vi "Change Waveform.vi"(8 "error in":errorcluster, 10 "Waveforms UI Ctrl Ref":T2, 11 "Waveform Meas Config Ctrl Ref":T1) -> (0 "error out":errorcluster)   [LabVIEW 2025, in "Fgen Script Mode UI.lvlib"]
uses:
  Fgen Script Mode UI.lvlib
  Typedef/Waveforms UI Ctrl Ref.ctl
  Typedef/Waveform Meas Config Ctrl Ref.ctl
  Typedef/Wfm Typedef.ctl
panel:
  in  "Auto Name?":bool=TRUE
  in  "Wfm Name in Script":string
  in  "Waveform Selection":i32(listbox)
  out "Selected Waveform Preview":waveform(dbl)(graph)
  in  "File Path":path
  in  "Cancel":bool
  in  "OK":bool
  # "* After configure the TDMS file path, select one waveform from the Waveform Selection to add and press OK."
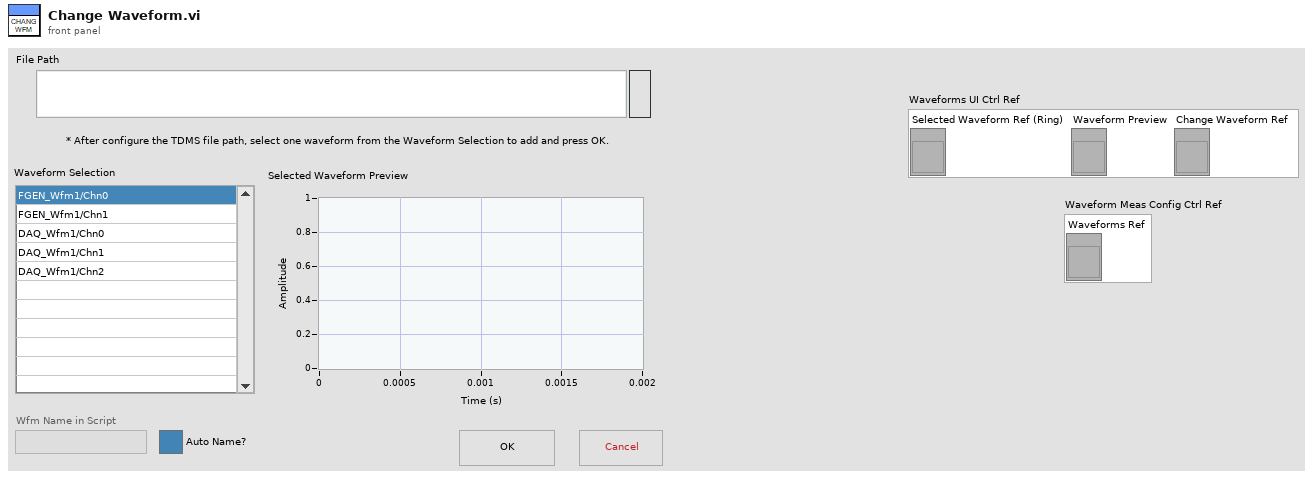
[diagram p1: front panel]
types:
  T1 = typedef "Fgen Script Mode UI.lvlib/Waveform Meas Config Ctrl Ref.ctl" = cluster{"Waveforms Ref":refnum<vi>}
  T2 = typedef "Fgen Script Mode UI.lvlib/Waveforms UI Ctrl Ref.ctl" = cluster{"Selected Waveform Ref (Ring)":refnum<vi>, "Waveform Preview":refnum<vi>, "Change Waveform Ref":refnum<vi>}
  T3 = typedef "Fgen Script Mode UI.lvlib/Wfm Typedef.ctl" = cluster{"Name":string, "Path":string, "Grp":string, "Chn":string}
  T4 = enum8{"Enabled", "Disabled", "Disabled and Grayed Out"}
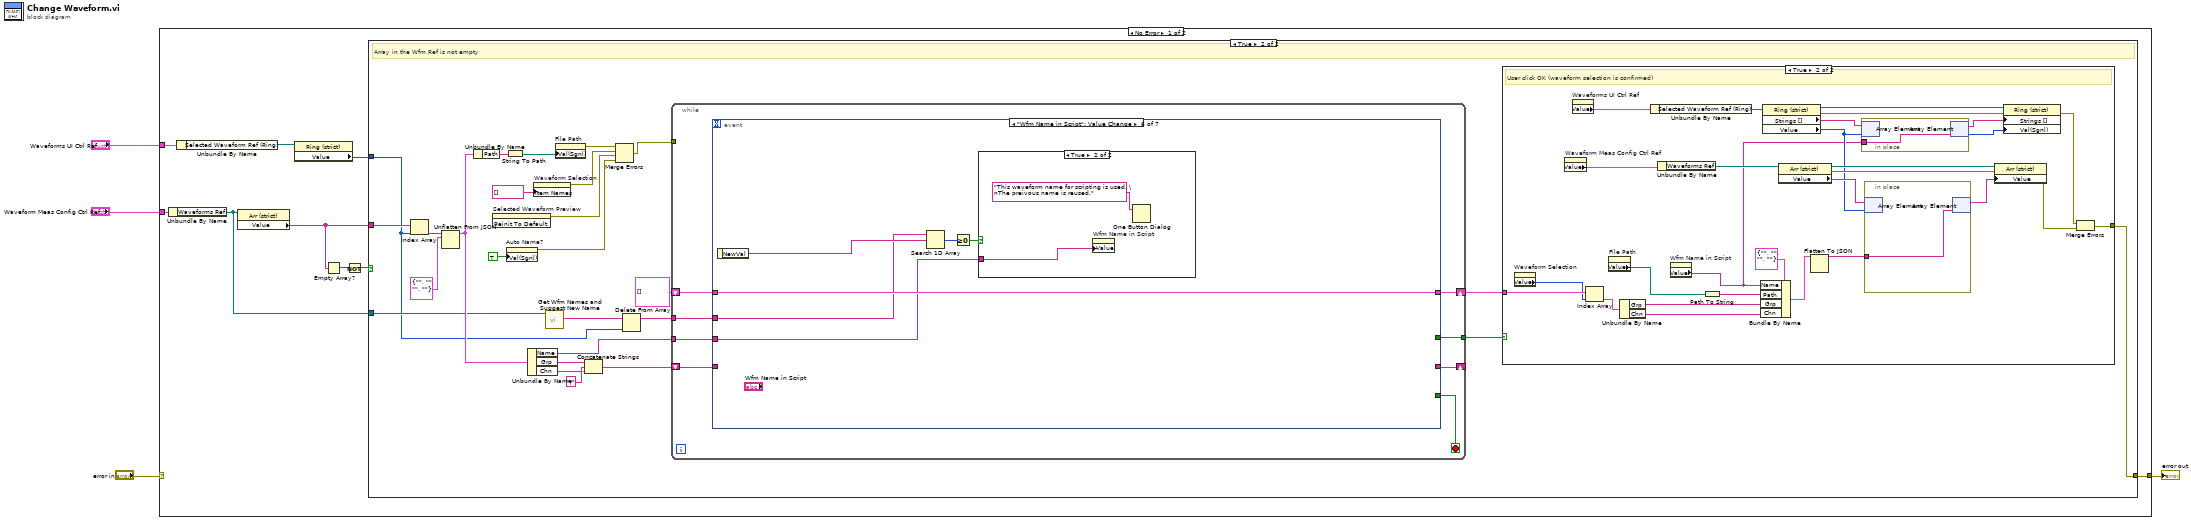
[diagram p0: block diagram]
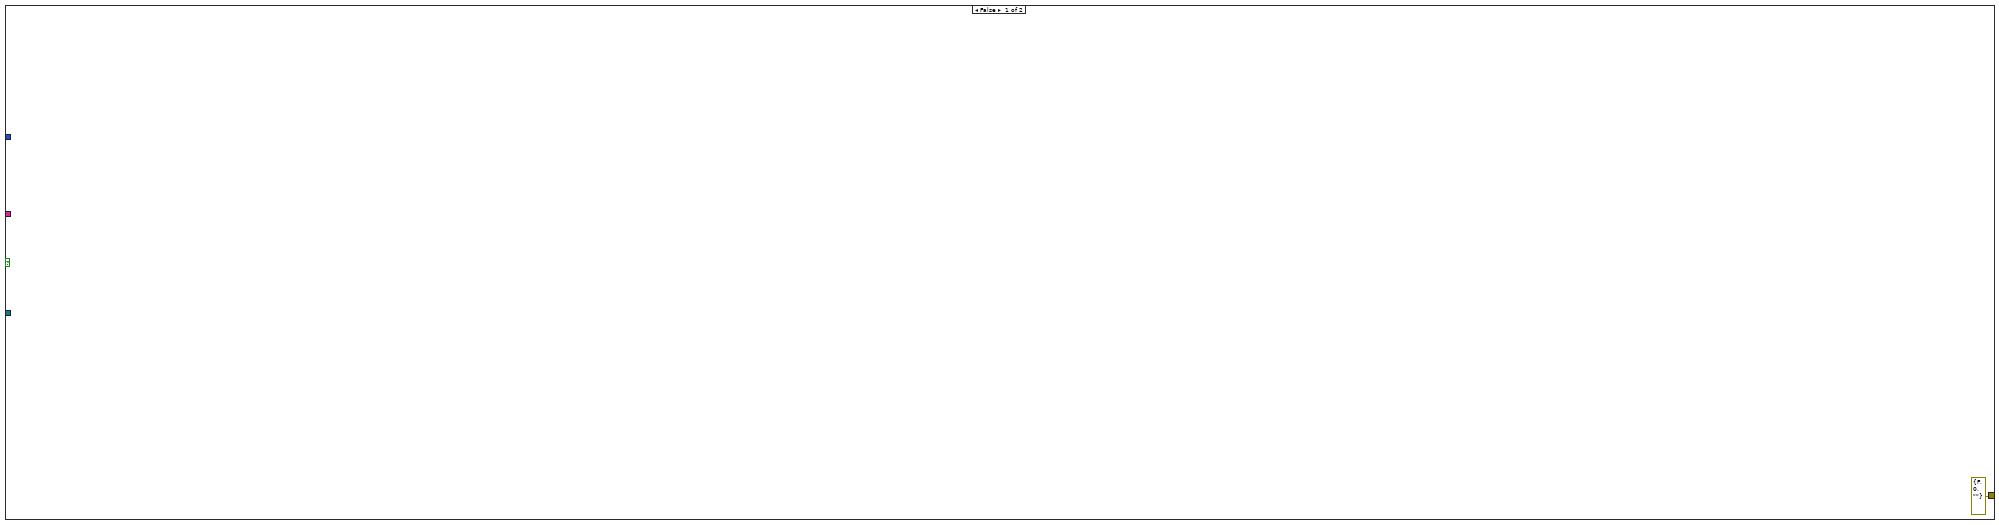
[diagram p2: hidden frame]
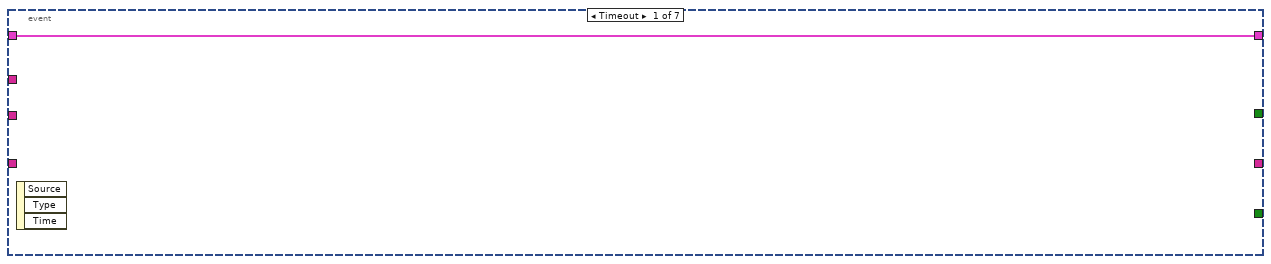
[diagram p4: hidden frame]
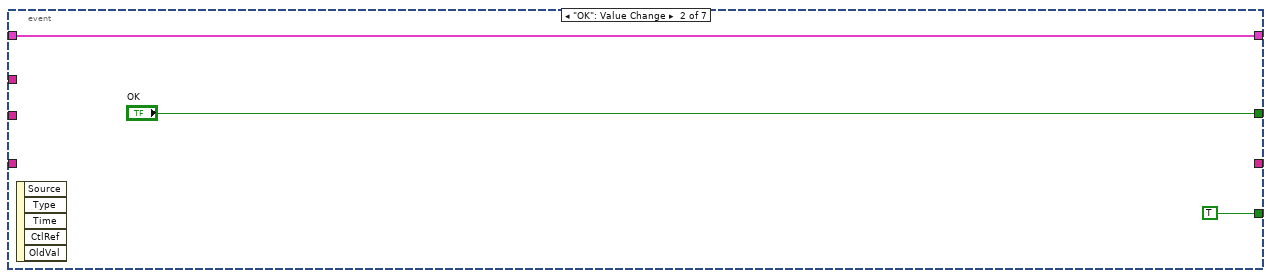
[diagram p5: hidden frame]
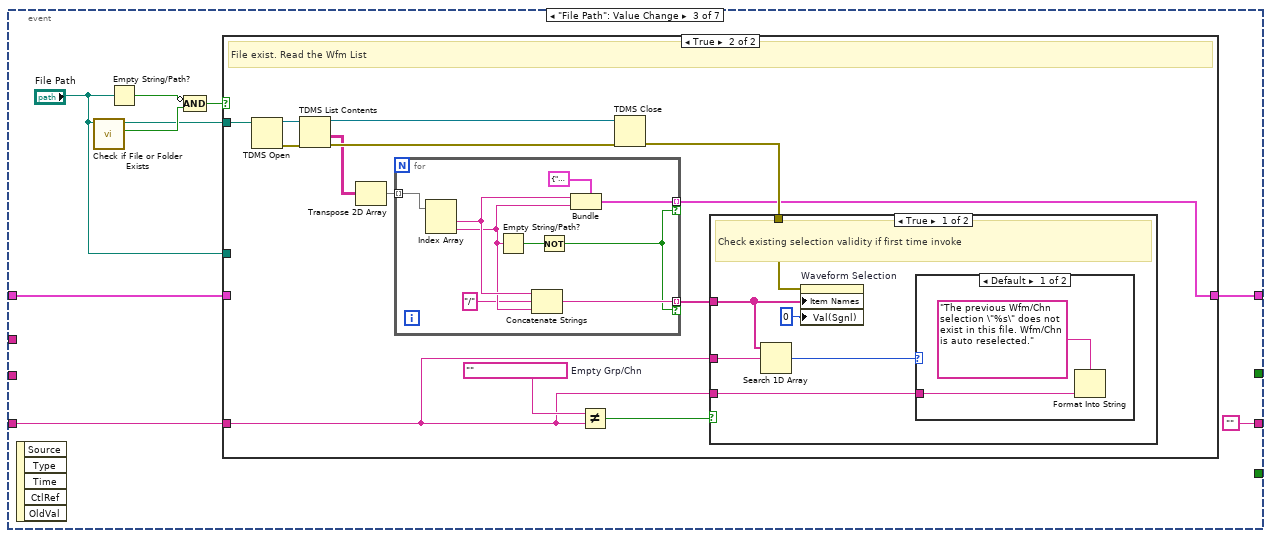
[diagram p6: hidden frame]
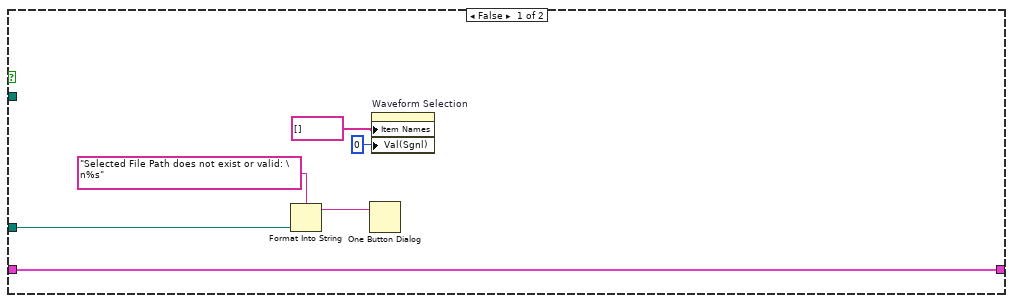
[diagram p7: hidden frame]
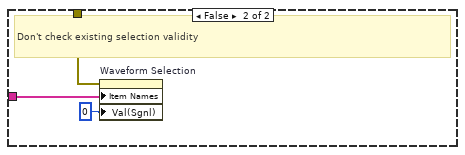
[diagram p9: hidden frame]
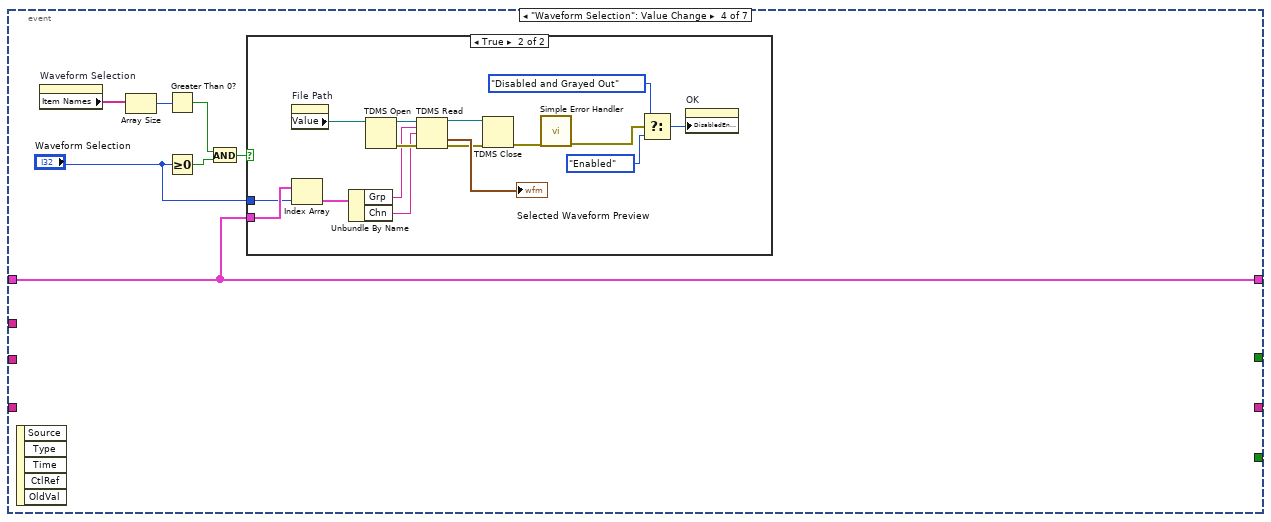
[diagram p10: hidden frame]
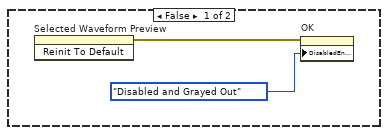
[diagram p11: hidden frame]
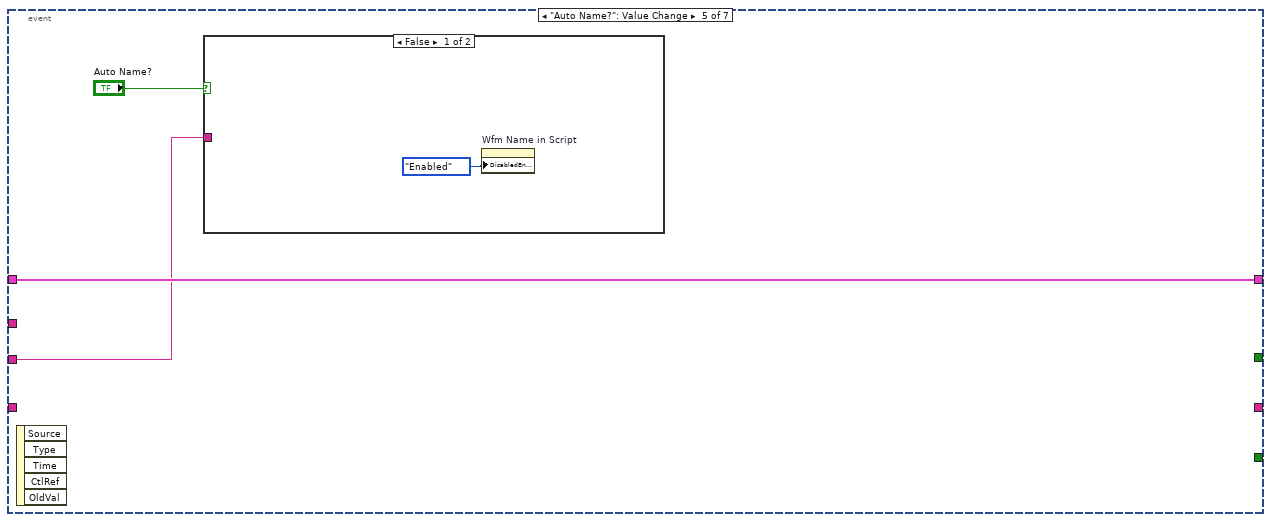
[diagram p12: hidden frame]
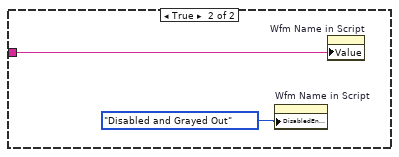
[diagram p13: hidden frame]
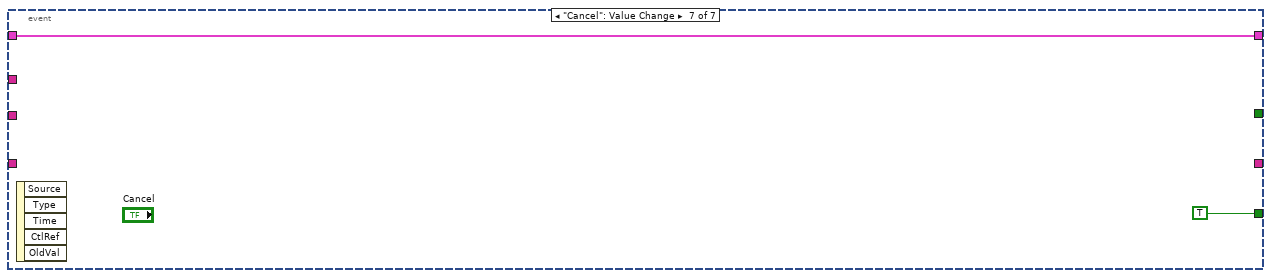
[diagram p15: hidden frame]
diagram:
  n1 = case shown="No Error" "error in" {
    selector: "error in" -> [_ w172]
    tunnel: [w13 w172] -> w3
    tunnel: "Waveforms UI Ctrl Ref" -> [w12 _]
    tunnel: "Waveform Meas Config Ctrl Ref" -> [w10 _]
    frame No Error {
      n2 = Unbundle By Name(w10) -> ("Waveforms Ref"=w7:refnum<vi>)
      n3 = Unbundle By Name(w12) -> ("Selected Waveform Ref (Ring)"=w11:refnum<vi>)
      n4 = property class="Arr (strict)"(reference=w7) -> ("Value"=w9:string[])  [unwired: 1 in, 2 out]
      n5 = property class="Ring (strict)"(reference=w11) -> ("Value"=w6:u16)  [unwired: 1 in, 2 out]
      n6 = Empty Array?(array=w9) -> (empty?=w8:bool)
      n7 = Not(x=w8) -> (.not. x?=w5:bool)
      n8 = case shown="True" w5 {
        tunnel: [errorcluster {"status"=FALSE, "code"=0, "source"=""} ("error IO") w32] -> w13
        tunnel: w9 -> [_ w29]
        tunnel: w7 -> [_ w19]
        tunnel: w6 -> [_ w17]
        frame False {
        }
        frame True {
          # "Array in the Wfm Ref is not empty"
          n9 = Index Array(array=w29, index=w17) -> (element=w27:string)
          n10 = Unflatten From JSON(JSON string=w27, type and defaults=T3 {"Name"="", "Path"="", "Grp"="", "Chn"=""} ("Waveform")) -> (value=w24:T3)  [unwired: 5 in, 1 out]
          n11 = Unbundle By Name(w24) -> ("Path"=w26:string)
          n12 = invoke on="Selected Waveform Preview" class="WFGraph (strict)" method="Reinit To Default"() -> (error out=w35:errorcluster)  [unwired: 3 in, 2 out]
          n13 = String To Path(string=w26) -> (path=w25:path)
          n14 = property on="Auto Name?" class="Bool (strict)"("Val(Sgnl)"=TRUE ("Value (Signaling)")) -> (error out=w31:errorcluster)  [unwired: 2 in, 1 out]
          n15 = Unbundle By Name(w24) -> ("Name"=w15:string, "Grp"=w22:string, "Chn"=w21:string)
          n16 = property on="Waveform Selection" class="LstBox (strict)"("Item Names"=string[] []) -> (error out=w36:errorcluster)  [unwired: 2 in, 1 out]
          n17 = call "Get Wfm Names and Suggest New Name.vi"("Wfm Ref In"=w19) -> ("Wfm Names"=w18:string[])  [unwired: 7 in, 3 out]
          n18 = property on="File Path" class="Path"("Val(Sgnl)"=w25) -> (error out=w39:errorcluster)  [unwired: 2 in, 1 out]
          n19 = Concatenate Strings(w22, "/" ("string"), w21) -> (w20:string)
          n20 = Merge Errors(w39, w36, w35, w31) -> (w37:errorcluster)
          n21 = Delete From Array(array=w18, index=w17) -> (array with subset deleted=w16:string[])  [unwired: 1 in, 1 out]
          n22 = while {
            tunnel: w37 -> [_]
            shift-right: [w77] -> w33
            shift-left: cluster{"Grp":string, "Chn":string}[] [] -> [w76]
            tunnel: [w75] -> w34
            shift-right: [w73] -> _
            shift-left: w20 -> [w74]
            tunnel: w16 -> [w72]
            tunnel: w15 -> [w71]
            stop <- w78 stop-if-true
            n23 = event shown="[5] \"Wfm Name in Script\": Value Change" {
              selector: _ -> [_ _ _ _ _ _ _]
              dyn-events: _ -> [_ _ _ _ _ _ _]
              timeout: _ -> [_ _ _ _ _ _ _]
              tunnel: [_ "OK" _ _ _ _ _] -> w75
              tunnel: [_ TRUE _ _ _ _ TRUE] -> w78
              tunnel: [w79 w80 w87 w132 w158 w167 w170] -> w77
              tunnel: w76 -> [w79 w80 w86 w132 w158 w167 w170]
              tunnel: w74 -> [_ _ w84 _ _ _ _]
              tunnel: [_ _ "" _ _ _ _] -> w73
              tunnel: w72 -> [_ _ _ _ _ w162 _]
              tunnel: w71 -> [_ _ _ _ w156 w163 _]
              event Timeout {
                n24 = event-data() -> ()  [unwired: 1 in, 3 out]
              }
              event "OK": Value Change {
                n25 = event-data() -> ()  [unwired: 1 in, 5 out]
              }
              event "File Path": Value Change {
                n26 = event-data() -> ()  [unwired: 1 in, 5 out]
                n27 = call <vilib>:"Check if File or Folder Exists.vi"("path"="File Path") -> ("file or folder exists?"=w90:bool, "dup path"=w88:path)  [unwired: 8 in, 1 out]
                n28 = Empty String/Path?(string/path="File Path") -> (empty?=w91:bool)
                n29 = Compound Arithmetic op=AND(invert w91, w90) -> (w89:bool)
                n30 = case shown="True" w89 {
                  tunnel: w88 -> [_ w110]
                  tunnel: [w97 w101] -> w87
                  tunnel: w86 -> [w97 _]
                  tunnel: "File Path" -> [w92 _]
                  tunnel: w84 -> [_ w98]
                  frame False {
                    n31 = Format Into String(format string="Selected File Path does not exist or valid: \n%s" ("message"), w92) -> (resulting string=w94:string)  [unwired: 2 in, 1 out]
                    n32 = One Button Dialog(message=w94) -> ()  [unwired: 1 in, 1 out]
                    n33 = property on="Waveform Selection" class="LstBox (strict)"("Item Names"=string[] [], "Val(Sgnl)"=0 ("Waveform Selection")) -> ()  [unwired: 2 in, 2 out]
                  }
                  frame True {
                    w100 = ""  # Empty Grp/Chn
                    # "File exist. Read the Wfm List"
                    n34 = TDMS Open(11:w110) -> (0:w109:errorcluster, 3:w108:refnum<k34>)  [unwired: 6 in]
                    n35 = TDMS List Contents(4:w109, 7:w108) -> (0:w106:errorcluster, 1:w104:string[][], 3:w107:refnum<k34>)  [unwired: 1 in, 1 out]
                    n36 = Transpose 2D Array(2D array=w104) -> (transposed array=w105:string[][])
                    n37 = for {
                      tunnel: w105 -> [w130] mode=indexing
                      tunnel: [w127] -> w101 mode=indexing if=w122
                      tunnel: [w123] -> w103 mode=indexing if=w122
                      n38 = Index Array(array=w130) -> (element #1=w126:string, element #2=w125:string)  [unwired: 2 in]
                      n39 = Empty String/Path?(string/path=w125) -> (empty?=w129:bool)
                      n40 = Concatenate Strings(w126, "/" ("string"), w125) -> (w123:string)
                      n41 = Not(x=w129) -> (.not. x?=w122:bool)
                      n42 = Bundle(cluster=cluster{"Grp":string, "Chn":string} {"Grp"="", "Chn"=""} ("output cluster"), "Grp"=w126, "Chn"=w125) -> (w127:cluster{"Grp":string, "Chn":string})
                    }
                    n43 = Not Equal?(x=w100, y=w98) -> (x != y?=w99:bool)
                    n44 = TDMS Close(8:w106, 11:w107) -> (0:w102:errorcluster)  [unwired: 1 out]
                    n45 = case shown="True" w99 {
                      tunnel: w103 -> [w113 w121]
                      tunnel: w102 -> [w116 w120]
                      tunnel: w98 -> [w114 _]
                      tunnel: w98 -> [w111 _]
                      frame True {
                        # "Check existing selection validity if first time invoke"
                        n46 = Search 1D Array(1D array=w113, element=w114) -> (index of element=w112:i32)  [unwired: 1 in]
                        n47 = property on="Waveform Selection" class="LstBox (strict)"(error in=w116, "Item Names"=w113, "Val(Sgnl)"=0 ("Waveform Selection")) -> ()  [unwired: 1 in, 2 out]
                        n48 = case shown="Default" w112 {
                          tunnel: w111 -> [w117 _]
                          frame Default {
                            n49 = Format Into String(format string="The previous Wfm/Chn selection \"%s\" does not exist in this file. Wfm/Chn is auto reselected.", w117) -> ()  [unwired: 2 in, 2 out]
                          }
                          frame 0.. {
                          }
                        }
                      }
                      frame False {
                        # "Don't check existing selection validity"
                        n50 = property on="Waveform Selection" class="LstBox (strict)"(error in=w120, "Item Names"=w121, "Val(Sgnl)"=0 ("Waveform Selection")) -> ()  [unwired: 1 in, 2 out]
                      }
                    }
                  }
                }
              }
              event "Waveform Selection": Value Change {
                n51 = event-data() -> ()  [unwired: 1 in, 5 out]
                n52 = property on="Waveform Selection" class="LstBox (strict)"() -> ("Item Names"=w136:string[])  [unwired: 2 in, 2 out]
                n53 = Array Size(array=w136) -> (size(s)=w135:i32)
                n54 = Greater Than 0?(x=w135) -> (x > 0?=w133:bool)
                n55 = Greater Or Equal To 0?(x="Waveform Selection") -> (x >= 0?=w137:bool)
                n56 = And(x=w133, y=w137) -> (x .and. y?=w134:bool)
                n57 = case shown="True" w134 {
                  tunnel: w132 -> [_ w154]
                  tunnel: "Waveform Selection" -> [_ w153]
                  frame False {
                    n58 = invoke on="Selected Waveform Preview" class="WFGraph (strict)" method="Reinit To Default"() -> (error out=w139:errorcluster)  [unwired: 3 in, 2 out]
                    n59 = property on="OK" class="Bool"(error in=w139, "DisabledEnum"=T4."Disabled and Grayed Out" ("Disabled")) -> ()  [unwired: 1 in, 2 out]
                  }
                  frame True {
                    n60 = property on="File Path" class="Path"() -> ("Value"=w155:path)  [unwired: 2 in, 2 out]
                    n61 = Index Array(array=w154, index=w153) -> (element=w150:cluster{"Grp":string, "Chn":string})
                    n62 = Unbundle By Name(w150) -> ("Grp"=w149:string, "Chn"=w148:string)
                    n63 = TDMS Open(11:w155) -> (0:w151:errorcluster, 3:w152:refnum<k34>)  [unwired: 6 in]
                    n64 = TDMS Read(0:w152, 5:w149, 7:w148, 11:w151) -> (4:w146:refnum<k34>, 10:→"Selected Waveform Preview":waveform(dbl), 15:w145:errorcluster)  [unwired: 4 in, 3 out]
                    n65 = TDMS Close(8:w145, 11:w146) -> (0:w144:errorcluster)  [unwired: 1 out]
                    n66 = call <vilib>:"Simple Error Handler.vi"("error in (no error)"=w144) -> ("error out"=w143:errorcluster)  [unwired: 4 in, 4 out]
                    n67 = Select(t=T4."Disabled and Grayed Out" ("Disabled"), s=w143, f=T4."Enabled" ("Disabled")) -> (s? t:f=w140:T4)
                    n68 = property on="OK" class="Bool"("DisabledEnum"=w140) -> ()  [unwired: 2 in, 2 out]
                  }
                }
              }
              event "Auto Name?": Value Change {
                n69 = event-data() -> ()  [unwired: 1 in, 5 out]
                n70 = case shown="False" "Auto Name?" {
                  tunnel: w156 -> [_ w160]
                  frame False {
                    n71 = property on="Wfm Name in Script" class="Str"("DisabledEnum"=T4."Enabled" ("Disabled")) -> ()  [unwired: 2 in, 2 out]
                  }
                  frame True {
                    n72 = property on="Wfm Name in Script" class="Str"("DisabledEnum"=T4."Disabled and Grayed Out" ("Disabled")) -> ()  [unwired: 2 in, 2 out]
                    n73 = property on="Wfm Name in Script" class="Str"("Value"=w160) -> ()  [unwired: 2 in, 2 out]
                  }
                }
              }
              event "Wfm Name in Script": Value Change {
                n74 = event-data() -> ("NewVal"=w166:string)  [unwired: 1 in]
                n75 = Search 1D Array(1D array=w162, element=w166) -> (index of element=w165:i32)  [unwired: 1 in]
                n76 = Greater Or Equal To 0?(x=w165) -> (x >= 0?=w164:bool)
                n77 = case shown="True" w164 {
                  tunnel: w163 -> [_ w168]
                  frame False {
                  }
                  frame True {
                    n78 = property on="Wfm Name in Script" class="Str"("Value"=w168) -> ()  [unwired: 2 in, 2 out]
                    n79 = One Button Dialog(message="This waveform name for scripting is used. \nThe preivous name is reused.") -> ()  [unwired: 1 in, 1 out]
                  }
                }
              }
              event "Cancel": Value Change {
                n80 = event-data() -> ()  [unwired: 1 in, 5 out]
              }
            }
          }
          n81 = case shown="True" w34 {
            tunnel: w33 -> [_ w68]
            tunnel: [_ w56] -> w32
            frame False {
            }
            frame True {
              # "User click OK (waveform selection is confirmed)"
              n82 = property on="Waveform Selection" class="LstBox (strict)"() -> ("Value"=w67:i32)  [unwired: 2 in, 2 out]
              n83 = property on="Waveform Meas Config Ctrl Ref" class="Clust (strict)"() -> ("Value"=w51:T1)  [unwired: 2 in, 2 out]
              n84 = property on="Waveforms UI Ctrl Ref" class="Clust (strict)"() -> ("Value"=w52:T2)  [unwired: 2 in, 2 out]
              n85 = Index Array(array=w68, index=w67) -> (element=w53:cluster{"Grp":string, "Chn":string})
              n86 = property on="File Path" class="Path"() -> ("Value"=w64:path)  [unwired: 2 in, 2 out]
              n87 = Unbundle By Name(w53) -> ("Grp"=w63:string, "Chn"=w62:string)
              n88 = Unbundle By Name(w52) -> ("Selected Waveform Ref (Ring)"=w59:refnum<vi>)
              n89 = Unbundle By Name(w51) -> ("Waveforms Ref"=w61:refnum<vi>)
              n90 = property on="Wfm Name in Script" class="Str"() -> ("Value"=w42:string)  [unwired: 2 in, 2 out]
              n91 = Path To String(path=w64) -> (string=w65:string)
              n92 = Bundle By Name(cluster=T3 {"Name"="", "Path"="", "Grp"="", "Chn"=""} ("Waveform"), "Name"=w42, "Path"=w65, "Grp"=w63, "Chn"=w62) -> (w60:T3)
              n93 = property class="Ring (strict)"(reference=w59) -> (reference out=w46:refnum<vi>, error out=w57:errorcluster, "Strings []"=w45:string[], "Value"=w44:u16)  [unwired: 1 in]
              n94 = property class="Arr (strict)"(reference=w61) -> (reference out=w55:refnum<vi>, error out=w54:errorcluster, "Value"=w50:string[])  [unwired: 1 in]
              n95 = Flatten To JSON(anything=w60) -> (JSON string=w49:string)  [unwired: 2 in, 1 out]
              n96 = in-place {
                in-place-border: w42 -> [w69]
                n97 = in-place-array #1(w45, w44) -> ()  [unwired: 1 out]
                n98 = in-place-array #1(w69) -> (w43:string[], w41:i32)
              }
              n99 = in-place {
                in-place-border: w49 -> [w70]
                n100 = in-place-array #2(w50, w44) -> ()  [unwired: 1 out]
                n101 = in-place-array #2(w70) -> (w48:string[])  [unwired: 1 out]
              }
              n102 = property class="Arr (strict)"(reference=w55, error in=w54, "Value"=w48) -> (error out=w58:errorcluster)  [unwired: 1 out]
              n103 = property class="Ring (strict)"(reference=w46, error in=w57, "Strings []"=w43, "Val(Sgnl)"=w41) -> (error out=w47:errorcluster)  [unwired: 1 out]
              n104 = Merge Errors(w47, w58) -> (w56:errorcluster)
            }
          }
        }
      }
    }
    frame Error {
    }
  }
  "error out" <- w3
